vi "Tag Names.vi"(11 "State in":T2={"State"=enum."Idle", "Start Time"=timestamp(0 s since 1904-01-01), "Configuration"={"Cycle Period"=0.0, "Ismatech"={"VISA resource name"="", "Simulated?"=FALSE, "Pump Number"=1.0, "Reverse?"=FALSE}, "Masterflex"={"VISA resource name"="", "Simulated?"=FALSE, "Pump Number"=1.0, "Reverse?"=FALSE}, "Mettler"={"VISA resource name"="", "Simulated?"=FALSE}, "Bronkhorst M13 Flow Meter"={"VISA resource name"="", "Simulated?"=FALSE, "Smoothing Steps"=1}, "PID 2 Parameters"={"Input Device"=enum."Bronkhorst M13", "Output Device"=enum."Ismatec ISM 831C", "Setpoint"=0.0, "PID gains"={"proportional gain (Kc)"=1.0, "integral time (Ti, min)"=0.01, "derivative time (Td, min)"=0.0}}, "Manual Entry"=0.0, "Auto?"=TRUE, "PID range"={"PID High"=100.0, "PID Low"=0.0, "High Warning"=100.0}, "Tacmina Settings"={"Analog DAQ Task"="", "Digital DAQ Task"=""}, "KNF SIMDOS Settings"={"VISA resource name"="", "Simulated?"=TRUE}, "ASIA Pump C"={"ASIA Pump #"=0, "channel"=0, "Simulated"=FALSE}, "VICI Settings"={"VISA resource name"="", "Pump ID"="", "Pump Head Vol"=0.0, "Reverse?"=FALSE, "Simulated?"=FALSE}, "FLOM Settings"={"VISA resource name"="", "Simulated?"=TRUE, "Pump Number"=0.0}, "SSI PR/LD Settings"={"VISA resource name"="", "Simulated?"=FALSE}, "Masterflex 75211 Settings"={"Analog DAQ Task"="", "Digital DAQ Task"=""}, "SSI P40 Settings"={"VISA resource name"="", "Simulated?"=TRUE}, "Ismatech 3 Channel Settings"={"VISA resource name"="", "Pump Number"=1, "Channel Number"=0, "Simulated?"=TRUE, "Reverse?"=FALSE}, "Bronkhorst M14 Settings"={"VISA resource name"="", "Simulated?"=FALSE, "Smoothing Steps"=1}, "Reset Totalizer"=FALSE, "Input Num Alarm Settings"=[], "Control Type"=enum."g/min", "Front End Display Options"={"Temperature"=TRUE, "Scale Grams"=FALSE, "Density"=TRUE, "Flow (g/min)"=FALSE, "Flow (ml/min)"=TRUE, "PSIG"=TRUE, "Total Grams"=TRUE, "Updated"=TRUE}}, "Current Time"=timestamp(0 s since 1904-01-01), "PID 1 Parameters"={"Setpoint"=0.0, "PID gains"={"proportional gain (Kc)"=1.0, "integral time (Ti, min)"=0.01, "derivative time (Td, min)"=0.0}}, "First Iteration"=FALSE, "Data"={"Flowmeter (g/min)"=0.0, "Flowmeter (ml/min)"=0.0, "Density"=0.0, "FL Temp"=0.0, "Scale Output (g)"=0.0, "Scale Rate of Change (g/min)"=0.0, "PID 1 Output"=0.0, "PID 2 Process Variable"=0.0, "PID 2 output"=0.0, "Pump Flow"=0.0, "Pump Pressure"=0.0, "Totalized Value"=0.0}, "Process Name"="", "Pump On?"=enum."Off", "Input Error"=FALSE, "Output Error"=FALSE, "Log Started"=FALSE, "PID Overshoot"=FALSE, "Current Setpoint"=0.0} {"PID 1 Parameters"."PID gains"."derivative time (Td, min)" format="%.3f"; "PID 1 Parameters"."PID gains"."integral time (Ti, min)" format="%.3f"; "PID 1 Parameters"."PID gains"."proportional gain (Kc)" format="%.3f"; "Configuration"."Bronkhorst M14 Settings"."Smoothing Steps" min=1 step=1; "Configuration"."Ismatech 3 Channel Settings"."Channel Number" min=0 max=3; "Configuration"."Ismatech 3 Channel Settings"."Pump Number" min=1; "Configuration"."PID range"."PID Low" min=0.0 max=100.0 format="%.2f"; "Configuration"."PID range"."PID High" format="%.2f"; "Configuration"."PID 2 Parameters"."PID gains"."derivative time (Td, min)" format="%.3f"; "Configuration"."PID 2 Parameters"."PID gains"."integral time (Ti, min)" format="%.3f"; "Configuration"."PID 2 Parameters"."PID gains"."proportional gain (Kc)" format="%.3f"; "Configuration"."Bronkhorst M13 Flow Meter"."Smoothing Steps" min=1 step=1; "Configuration"."ASIA Pump C"."channel" min=0 max=1 step=1; "Configuration"."Ismatech"."Pump Number" min=1.0 max=20.0 step=1.0; "Configuration"."Masterflex"."Pump Number" min=1.0 max=20.0 step=1.0}) -> (0 "All  Flow Meter Tags":string[](array[string]), 1 "All  Scale Tags":string[](array[string]), 3 "Feed Module Tag Names":T1, 4 "All Boolean Tags":string[](array[string]), 5 "All  Numeric Tags":string[](array[string]))   [LabVIEW 2018, in "Feed Module.lvlib" / "Feed Module Engine.lvlib"]
uses:
  Feed Module Engine.lvlib
  State Cluster.ctl
  State Enum.ctl
  Feed Module/Controls/Feed Module Settings Cluster.ctl
  Ismatec ISM 831C/Controls/Ismatech ISM831C Settings Cluster.ctl
  Masterflex 7550-30/Controls/Settings Cluster.ctl
  Mettler Toledo/Controls/Settings Cluster.ctl
  Bronkhorst M13 Flow Meter/Settings Cluster.ctl
  PID 2 Parameters Cluster.ctl
  PID Input Enum.ctl
  PID 2 Output Enum.ctl
  Tacmina QI/Tacmina QI DAQ Setting.ctl
  KNF Pump/Settings Cluster plus SIMDOS.ctl
  ASIA Pump/Pump Settings.ctl
  VICI M50 Party Mode/Settings Cluster.ctl
  FLOM Pump/Settings Cluster.ctl
  SSI PR Class/SSI PR or LD Settings Cluster.ctl
  Masterflex 75211/Masterflex 75211 DAQ Setting.ctl
  SSI PR Class/SSI P40 Settings Cluster.ctl
  Ismatec 78001/Ismatec 4083.ctl
  Bronkhorst M14 Flow Meter/Settings Cluster.ctl
  Tag VIs/Numeric Alarm Settings Cluster.ctl
  PID 1 Parameters Cluster.ctl
  Feed Module/Controls/Feed Module Tag Names Cluster.ctl
  Feed Module/Feed Module.lvlib
  Ismatec ISM 831C/Ismatec ISM 831C.lvlib
  Masterflex 7550-30/Masterflex 7550-30.lvlib
  Mettler Toledo/Mettler Toledo.lvlib
  Bronkhorst M13 Flow Meter/Bronkhorst M13 Flow Meter.lvlib
  Tacmina QI/Tacmina QI.lvlib
  KNF Pump/KNF SIMDOS.lvlib
  ASIA Pump.lvlib
  VICI M50 Party Mode/VICI M6 M50 Party Mode.lvlib
  FLOM Pump/FLOM Pump.lvlib
  SSI PR Class/SSI PR or LD Pump.lvlib
  Masterflex 75211/Masterflex 75211.lvlib
  SSI PR Class/SSI P40 Pump.lvlib
  Ismatec 78001/Ismatec 4308.lvlib
  Bronkhorst M14 Flow Meter/Bronkhorst M14 Flow Meter.lvlib
panel:
  out "Pump Flow Tag":string
  out "PID 2 Out Tag":string
  out "Scale Tag":string
  # "Output Instruments"
  # "Input Instruments"
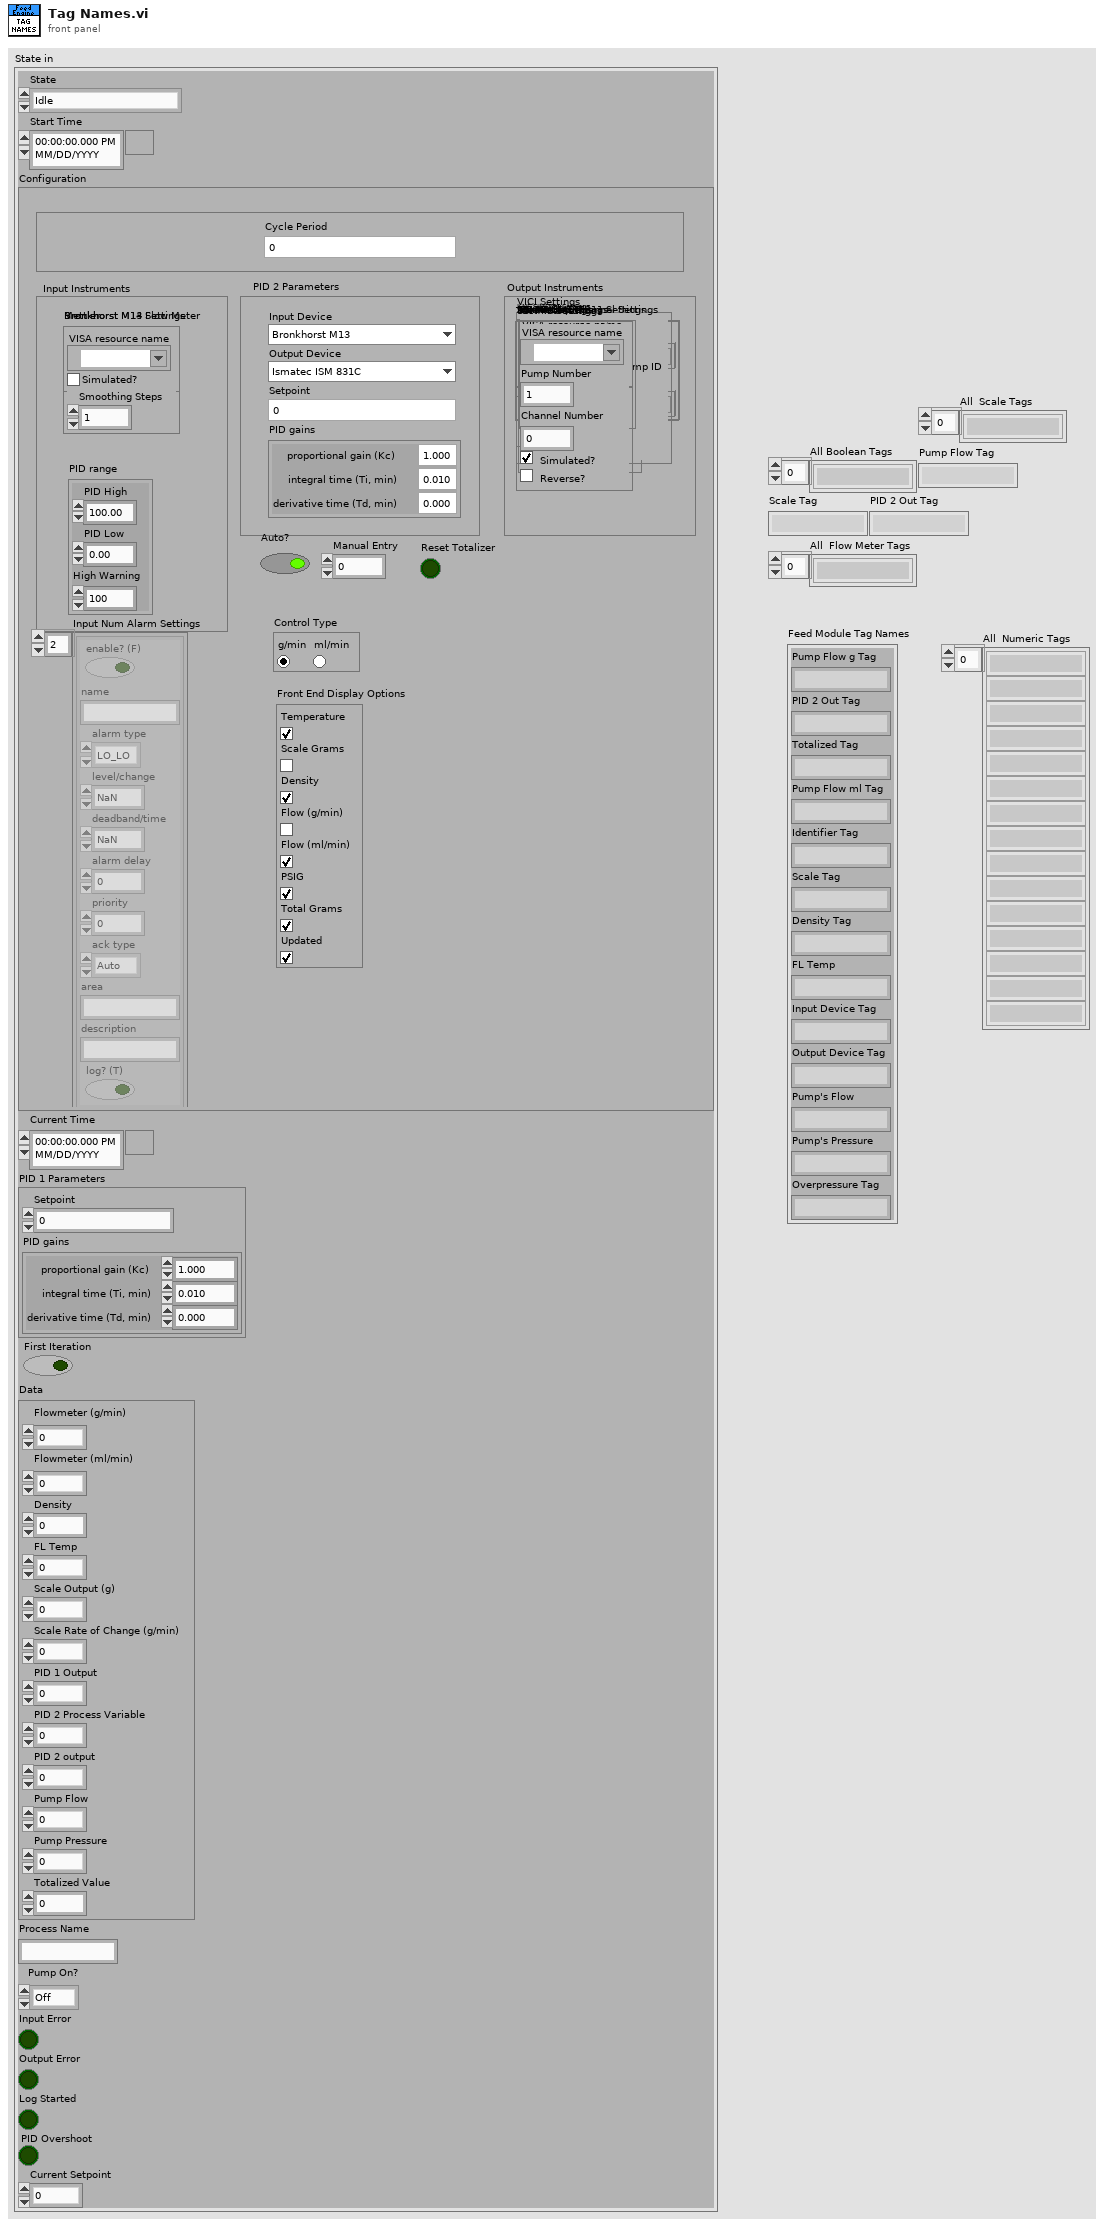
[diagram p1: front panel]
types:
  T1 = typedef "Feed Module.lvlib/Feed Module Tag Names Cluster.ctl" = cluster{"Pump Flow g Tag":string, "PID 2 Out Tag":string, "Totalized Tag":string, "Pump Flow ml Tag":string, "Identifier Tag":string, "Scale Tag":string, "Density Tag":string, "FL Temp":string, "Input Device Tag":string, "Output Device Tag":string, "Pump's Flow":string, "Pump's Pressure":string, "Overpressure Tag":string}
  T2 = typedef "Feed Module.lvlib/Feed Module Engine.lvlib/State Cluster.ctl" = cluster{"State":T3, "Start Time":timestamp, "Configuration":T4, "Current Time":timestamp, "PID 1 Parameters":T23, "First Iteration":bool, "Data":cluster{"Flowmeter (g/min)":dbl, "Flowmeter (ml/min)":dbl, "Density":dbl, "FL Temp":dbl, "Scale Output (g)":dbl, "Scale Rate of Change (g/min)":dbl, "PID 1 Output":dbl, "PID 2 Process Variable":dbl, "PID 2 output":dbl, "Pump Flow":dbl, "Pump Pressure":dbl, "Totalized Value":dbl}, "Process Name":string, "Pump On?":enum16{"Off", "On", "Not Initialized"}, "Input Error":bool, "Output Error":bool, "Log Started":bool, "PID Overshoot":bool, "Current Setpoint":dbl}
  T3 = typedef "Feed Module.lvlib/Feed Module Engine.lvlib/State Enum.ctl" = enum16{"Measuring", "Idle", "Paused"}
  T4 = typedef "Feed Module.lvlib/Feed Module Settings Cluster.ctl" = cluster{"Cycle Period":dbl, "Ismatech":T5, "Masterflex":T6, "Mettler":T7, "Bronkhorst M13 Flow Meter":T8, "PID 2 Parameters":T9, "Manual Entry":dbl, "Auto?":bool, "PID range":cluster{"PID High":dbl, "PID Low":dbl, "High Warning":dbl}, "Tacmina Settings":T12, "KNF SIMDOS Settings":T13, "ASIA Pump C":T14, "VICI Settings":T15, "FLOM Settings":T16, "SSI PR/LD Settings":T17, "Masterflex 75211 Settings":T18, "SSI P40 Settings":T19, "Ismatech 3 Channel Settings":T20, "Bronkhorst M14 Settings":T21, "Reset Totalizer":bool, "Input Num Alarm Settings":T22[], "Control Type":enum32{"g/min", "ml/min"}, "Front End Display Options":cluster{"Temperature":bool, "Scale Grams":bool, "Density":bool, "Flow (g/min)":bool, "Flow (ml/min)":bool, "PSIG":bool, "Total Grams":bool, "Updated":bool}}
  T5 = typedef "Ismatec ISM 831C.lvlib/Ismatech ISM831C Settings Cluster.ctl" = cluster{"VISA resource name":refnum<visa-resource-name>, "Simulated?":bool, "Pump Number":dbl, "Reverse?":bool}
  T6 = typedef "Masterflex 7550-30.lvlib/Settings Cluster.ctl" = cluster{"VISA resource name":refnum<visa-resource-name>, "Simulated?":bool, "Pump Number":dbl, "Reverse?":bool}
  T7 = typedef "Mettler Toledo.lvlib/Settings Cluster.ctl" = cluster{"VISA resource name":refnum<visa-resource-name>, "Simulated?":bool}
  T8 = typedef "Bronkhorst M13 Flow Meter.lvlib/Settings Cluster.ctl" = cluster{"VISA resource name":refnum<visa-resource-name>, "Simulated?":bool, "Smoothing Steps":i32}
  T9 = typedef "PID 2 Parameters Cluster.ctl" = cluster{"Input Device":T10, "Output Device":T11, "Setpoint":dbl, "PID gains":cluster{"proportional gain (Kc)":dbl, "integral time (Ti, min)":dbl, "derivative time (Td, min)":dbl}}
  T10 = typedef "PID Input Enum.ctl" = enum16{"Default", "Bronkhorst M13", "Bronkhorst M14", "Scale Rate of Change"}
  T11 = typedef "PID 2 Output Enum.ctl" = enum16{"Default", "Ismatec ISM 4308", "Ismatec ISM 831C", "Masterflex 7550-30", "VICI M6", "VICI M50", "Tacmina QI", "KNF SIMDOS", "ASIA Type C", "FLOM UI-22-11", "SSI PR/LD", "SSI P40", "Masterflex 75211-70"}
  T12 = typedef "Tacmina QI.lvlib/Tacmina QI DAQ Setting.ctl" = cluster{"Analog DAQ Task":refnum<k21>, "Digital DAQ Task":refnum<k21>}
  T13 = typedef "KNF SIMDOS.lvlib/Settings Cluster plus SIMDOS.ctl" = cluster{"VISA resource name":refnum<visa-resource-name>, "Simulated?":bool}
  T14 = typedef "ASIA Pump.lvlib/Pump Settings.ctl" = cluster{"ASIA Pump #":i32, "channel":i32, "Simulated":bool}
  T15 = typedef "VICI M6 M50 Party Mode.lvlib/Settings Cluster.ctl" = cluster{"VISA resource name":refnum<visa-resource-name>, "Pump ID":string, "Pump Head Vol":dbl, "Reverse?":bool, "Simulated?":bool}
  T16 = typedef "FLOM Pump.lvlib/Settings Cluster.ctl" = cluster{"VISA resource name":refnum<visa-resource-name>, "Simulated?":bool, "Pump Number":dbl}
  T17 = typedef "SSI PR or LD Pump.lvlib/SSI PR or LD Settings Cluster.ctl" = cluster{"VISA resource name":refnum<visa-resource-name>, "Simulated?":bool}
  T18 = typedef "Masterflex 75211.lvlib/Masterflex 75211 DAQ Setting.ctl" = cluster{"Analog DAQ Task":refnum<k21>, "Digital DAQ Task":refnum<k21>}
  T19 = typedef "SSI P40 Pump.lvlib/SSI P40 Settings Cluster.ctl" = cluster{"VISA resource name":refnum<visa-resource-name>, "Simulated?":bool}
  T20 = typedef "Ismatec 4308.lvlib/Ismatec 4083.ctl" = cluster{"VISA resource name":refnum<visa-resource-name>, "Pump Number":i16, "Channel Number":i16, "Simulated?":bool, "Reverse?":bool}
  T21 = typedef "Bronkhorst M14 Flow Meter.lvlib/Settings Cluster.ctl" = cluster{"VISA resource name":refnum<visa-resource-name>, "Simulated?":bool, "Smoothing Steps":i32}
  T22 = typedef "Numeric Alarm Settings Cluster.ctl" = cluster{"enable? (F)":bool, "name":string, "alarm type":enum16{"HI_HI", "HI", "LO", "LO_LO"}, "level/change":dbl, "deadband/time":dbl, "alarm delay":dbl, "priority":u32, "ack type":enum16{"Auto", "User", "None", "Each Occurrence"}, "area":string, "description":string, "log? (T)":bool}
  T23 = typedef "PID 1 Parameters Cluster.ctl" = cluster{"Setpoint":dbl, "PID gains":cluster{"proportional gain (Kc)":dbl, "integral time (Ti, min)":dbl, "derivative time (Td, min)":dbl}}
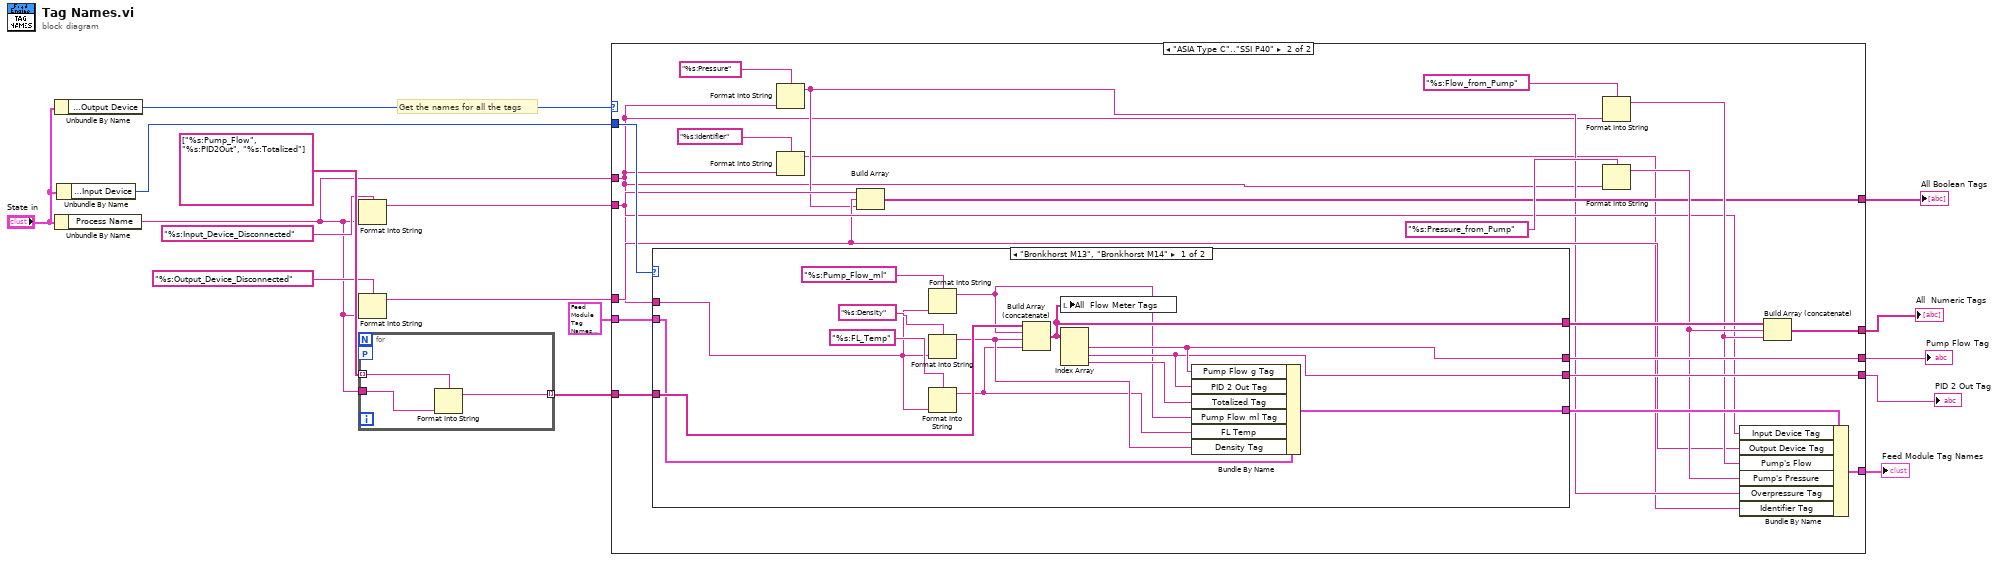
[diagram p0: block diagram]
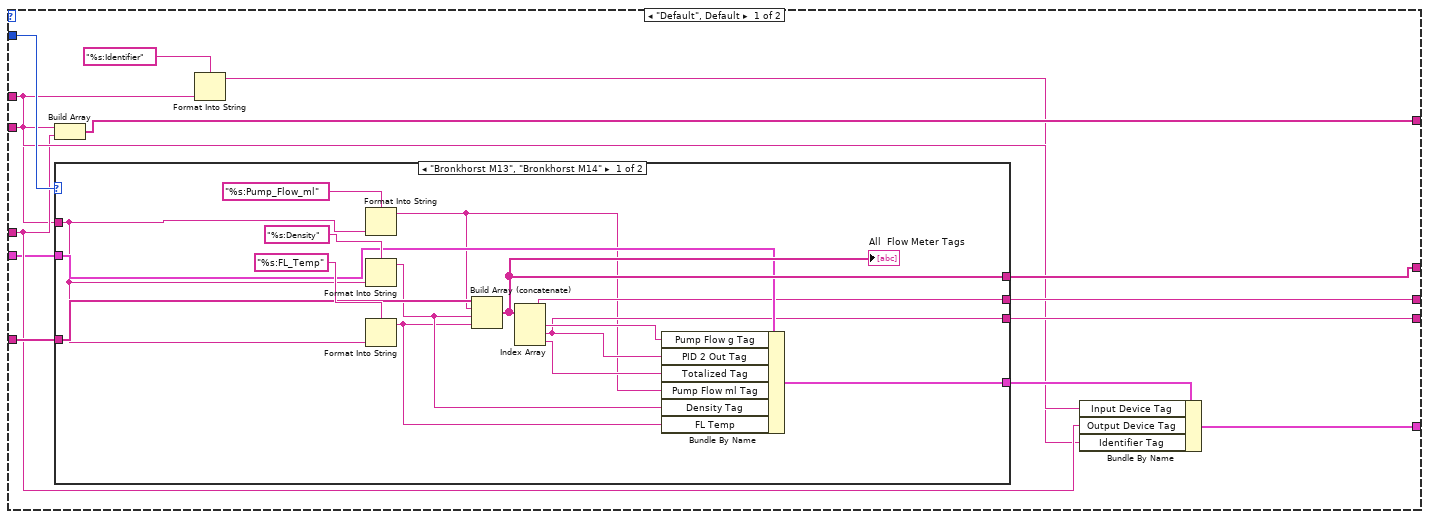
[diagram p2: hidden frame]
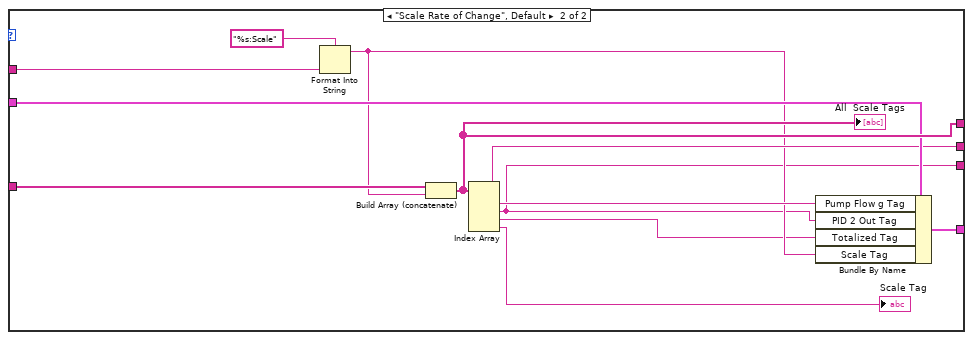
[diagram p3: hidden frame]
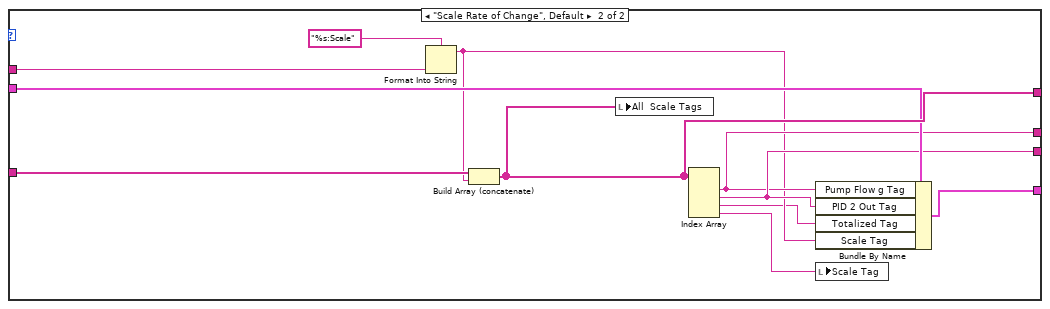
[diagram p4: hidden frame]
diagram:
  # "Get the names for all the tags"
  n1 = Unbundle By Name("State in") -> ("Configuration.PID 2 Parameters.Output Device"=w13:T11)
  n2 = Unbundle By Name("State in") -> ("Process Name"=w1:string)
  n3 = Unbundle By Name("State in") -> ("Configuration.PID 2 Parameters.Input Device"=w12:T10)
  n4 = Format Into String(format string="%s:Input_Device_Disconnected", w1) -> (resulting string=w4:string)  [unwired: 2 in, 1 out]
  n5 = Format Into String(format string="%s:Output_Device_Disconnected", w1) -> (resulting string=w3:string)  [unwired: 2 in, 1 out]
  n6 = for {
    tunnel: string[] ["%s:Pump_Flow", "%s:PID2Out", "%s:Totalized"] -> [w19] mode=indexing
    tunnel: w1 -> [w18]
    tunnel: [w17] -> w11 mode=indexing
    workers-P: _ -> [_]
    n7 = Format Into String(format string=w19, w18) -> (resulting string=w17:string)  [unwired: 2 in, 1 out]
  }
  n8 = case shown="\"ASIA Type C\"..\"SSI P40\"" w13 {
    tunnel: w1 -> [w22 w60]
    tunnel: w12 -> [w33 w77]
    tunnel: w11 -> [w32 w76]
    tunnel: [w31 w75] -> w10
    tunnel: [w30 w73] -> w7
    tunnel: [w29 w72] -> w8
    tunnel: [w28 w70] -> w6
    tunnel: w4 -> [w26 w66]
    tunnel: w3 -> [w25 w65]
    tunnel: [w24 w64] -> w5
    tunnel: T1 {"Pump Flow g Tag"="", "PID 2 Out Tag"="", "Totalized Tag"="", "Pump Flow ml Tag"="", "Identifier Tag"="", "Scale Tag"="", "Density Tag"="", "FL Temp"="", "Input Device Tag"="", "Output Device Tag"="", "Pump's Flow"="", "Pump's Pressure"="", "Overpressure Tag"=""} ("Feed Module Tag Names") -> [w20 w62]
    frame "Default", Default {
      n9 = Build Array(w26, w25) -> (w24:string[])
      n10 = case shown="\"Bronkhorst M13\", \"Bronkhorst M14\"" w33 {
        tunnel: w32 -> [w45 w58]
        tunnel: [w44 w55] -> w31
        tunnel: w22 -> [w34 w56]
        tunnel: [w42 w52] -> w29
        tunnel: [w41 w50] -> w30
        tunnel: w20 -> [w43 w54]
        tunnel: [w40 w53] -> w27
        frame "Bronkhorst M13", "Bronkhorst M14" {
          n11 = Format Into String(format string="%s:Pump_Flow_ml", w34) -> (resulting string=w35:string)  [unwired: 2 in, 1 out]
          n12 = Format Into String(format string="%s:Density", w34) -> (resulting string=w39:string)  [unwired: 2 in, 1 out]
          n13 = Format Into String(format string="%s:FL_Temp", w34) -> (resulting string=w38:string)  [unwired: 2 in, 1 out]
          n14 = Build Array (concatenate)(w45, w35, w39, w38) -> (w44:string[])
          "All  Flow Meter Tags" <- w44
          n15 = Index Array(array=w44) -> (element #1=w42:string, element #2=w41:string, element #3=w37:string)  [unwired: 3 in]
          n16 = Bundle By Name(cluster=w43, "Pump Flow g Tag"=w42, "PID 2 Out Tag"=w41, "Totalized Tag"=w37, "Pump Flow ml Tag"=w35, "Density Tag"=w39, "FL Temp"=w38) -> (w40:T1)
        }
        frame "Scale Rate of Change", Default {
          n17 = Format Into String(format string="%s:Scale", w56) -> (resulting string=w51:string)  [unwired: 2 in, 1 out]
          n18 = Build Array (concatenate)(w58, w51) -> (w55:string[])
          "All  Scale Tags" <- w55
          n19 = Index Array(array=w55) -> (element #1=w52:string, element #2=w50:string, element #3=w49:string, element #4=→"Scale Tag":string)  [unwired: 4 in]
          n20 = Bundle By Name(cluster=w54, "Pump Flow g Tag"=w52, "PID 2 Out Tag"=w50, "Totalized Tag"=w49, "Scale Tag"=w51) -> (w53:T1)
        }
      }
      n21 = Format Into String(format string="%s:Identifier", w22) -> (resulting string=w21:string)  [unwired: 2 in, 1 out]
      n22 = Bundle By Name(cluster=w27, "Input Device Tag"=w26, "Output Device Tag"=w25, "Identifier Tag"=w21) -> (w28:T1)
    }
    frame "ASIA Type C".."SSI P40" {
      n23 = case shown="\"Bronkhorst M13\", \"Bronkhorst M14\"" w77 {
        tunnel: w76 -> [w91 w104]
        tunnel: [w90 w101] -> w74
        tunnel: w60 -> [w80 w102]
        tunnel: [w88 w97] -> w72
        tunnel: [w87 w98] -> w73
        tunnel: w62 -> [w89 w100]
        tunnel: [w86 w99] -> w71
        frame "Bronkhorst M13", "Bronkhorst M14" {
          n24 = Format Into String(format string="%s:Pump_Flow_ml", w80) -> (resulting string=w81:string)  [unwired: 2 in, 1 out]
          n25 = Format Into String(format string="%s:Density", w80) -> (resulting string=w85:string)  [unwired: 2 in, 1 out]
          n26 = Format Into String(format string="%s:FL_Temp", w80) -> (resulting string=w84:string)  [unwired: 2 in, 1 out]
          n27 = Build Array (concatenate)(w91, w81, w85, w84) -> (w90:string[])
          n28 = local write "All  Flow Meter Tags"(w90) -> ()
          n29 = Index Array(array=w90) -> (element #1=w88:string, element #2=w87:string, element #3=w83:string)  [unwired: 3 in]
          n30 = Bundle By Name(cluster=w89, "Pump Flow g Tag"=w88, "PID 2 Out Tag"=w87, "Totalized Tag"=w83, "Pump Flow ml Tag"=w81, "FL Temp"=w84, "Density Tag"=w85) -> (w86:T1)
        }
        frame "Scale Rate of Change", Default {
          n31 = Format Into String(format string="%s:Scale", w102) -> (resulting string=w96:string)  [unwired: 2 in, 1 out]
          n32 = Build Array (concatenate)(w104, w96) -> (w101:string[])
          n33 = local write "All  Scale Tags"(w101) -> ()
          n34 = Index Array(array=w101) -> (element #1=w97:string, element #2=w98:string, element #3=w94:string, element #4=w95:string)  [unwired: 4 in]
          n35 = Bundle By Name(cluster=w100, "Pump Flow g Tag"=w97, "PID 2 Out Tag"=w98, "Totalized Tag"=w94, "Scale Tag"=w96) -> (w99:T1)
          n36 = local write "Scale Tag"(w95) -> ()
        }
      }
      n37 = Format Into String(format string="%s:Pressure", w60) -> (resulting string=w63:string)  [unwired: 2 in, 1 out]
      n38 = Format Into String(format string="%s:Identifier", w60) -> (resulting string=w59:string)  [unwired: 2 in, 1 out]
      n39 = Build Array(w66, w65, w63) -> (w64:string[])
      n40 = Format Into String(format string="%s:Flow_from_Pump", w60) -> (resulting string=w68:string)  [unwired: 2 in, 1 out]
      n41 = Format Into String(format string="%s:Pressure_from_Pump", w60) -> (resulting string=w69:string)  [unwired: 2 in, 1 out]
      n42 = Bundle By Name(cluster=w71, "Input Device Tag"=w66, "Output Device Tag"=w65, "Pump's Flow"=w68, "Pump's Pressure"=w69, "Overpressure Tag"=w63, "Identifier Tag"=w59) -> (w70:T1)
      n43 = Build Array (concatenate)(w74, w69, w68) -> (w75:string[])
    }
  }
  "All  Numeric Tags" <- w10
  "All Boolean Tags" <- w5
  "PID 2 Out Tag" <- w7
  "Pump Flow Tag" <- w8
  "Feed Module Tag Names" <- w6
